vi "autofocus calibrate.vi"() -> ()   [LabVIEW 2014]
uses:
  autofocus-globals.vi
  Stage Control/Stage SubVis/move stage.ctl
panel:
  out "Calibration curve":cluster{dbl[], ext[]}(graph)
  out "Cal. curve":cluster{ext[], dbl[]}
  out "Intensity OK":bool=TRUE
  in  "Error In":errorcluster
  out "Error Out":errorcluster
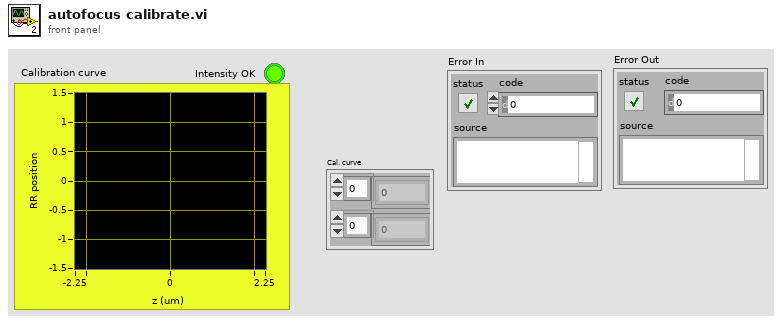
[diagram p1: front panel]
types:
  T1 = typedef "move stage.ctl" = cluster{"dx (um) (0 -> ignore)":ext, "dy (um) (0 -> ignore)":ext, "dz (um) (0 -> ignore)":ext, "Re-center x,y":bool, "Re-center z":bool, "x (um) (-1 -> ignore)":dbl, "y (um) (-1 -> ignore)":dbl, "z (um) (-1 -> ignore)":dbl}
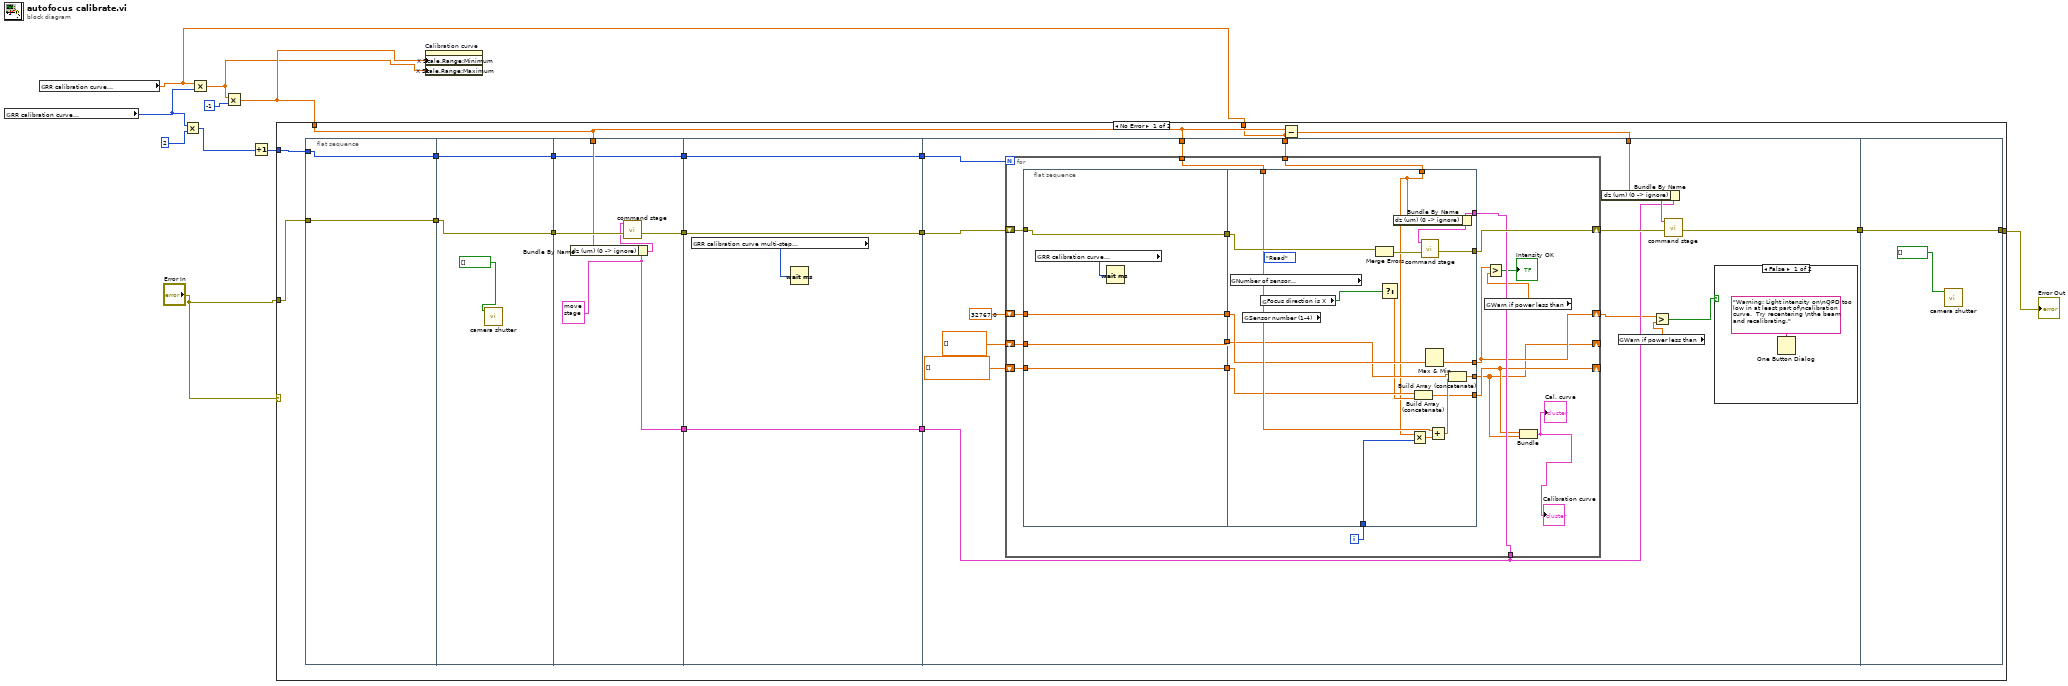
[diagram p0: block diagram]
diagram:
  n1 = global read "autofocus-globals.vi" "RR calibration curve\nhalf-width  (steps)"() -> (w6:u16)
  n2 = global read "autofocus-globals.vi" "RR calibration curve\nstep size (um)"() -> (w3:ext)
  n3 = Multiply(x=w6, y=2) -> (x*y=w5:i32)
  n4 = Multiply(x=w3, y=w6) -> (x*y=w1:ext)
  n5 = Multiply(x=w1, y=-1) -> (x*y=w2:ext)
  n6 = Increment(x=w5) -> (x+1=w4:i32)
  n7 = case shown="No Error" "Error In" {
    tunnel: "Error In" -> [w25 w103]
    tunnel: [w11 w103] -> w9
    tunnel: w2 -> [w15 _]
    tunnel: w4 -> [w27 _]
    tunnel: w3 -> [w14 _]
    frame No Error {
      n8 = flat-sequence {
        tunnel: w27 -> [w28]
        tunnel: [w29] -> w26
        tunnel: w25 -> [w29]
        tunnel: [w28] -> w19
        tunnel: w26 -> [w31]
        tunnel: [w31] -> w24
        tunnel: [w30] -> w20
        tunnel: w19 -> [w30]
        tunnel: w24 -> [w38]
        tunnel: w15 -> [w36]
        tunnel: [w37] -> w23
        tunnel: [w34] -> w22
        tunnel: [w33] -> w21
        tunnel: w20 -> [w33]
        tunnel: w23 -> [w42]
        tunnel: w22 -> [w41]
        tunnel: w21 -> [w39]
        tunnel: [w42] -> w18
        tunnel: [w41] -> w17
        tunnel: [w39] -> w16
        tunnel: w18 -> [w56]
        tunnel: w17 -> [w47]
        tunnel: w16 -> [w57]
        tunnel: w15 -> [w52]
        tunnel: w14 -> [w51]
        tunnel: w13 -> [w49]
        tunnel: [w46] -> w12
        tunnel: [w102] -> w11
        tunnel: w12 -> [w102]
        frame #0 {
        }
        frame #1 {
          n9 = call "camera shutter.vi"("Array"=bool[] []) -> ()  [unwired: 10 in, 1 out]
        }
        frame #2 {
          w34 = T1 {"dx (um) (0 -> ignore)"=0.0, "dy (um) (0 -> ignore)"=0.0, "dz (um) (0 -> ignore)"=0.0, "Re-center x,y"=FALSE, "Re-center z"=FALSE, "x (um) (-1 -> ignore)"=-1.0, "y (um) (-1 -> ignore)"=-1.0, "z (um) (-1 -> ignore)"=-1.0} ("Command Stage")
          n10 = Bundle By Name(cluster=w34, "dz (um) (0 -> ignore)"=w36) -> (w35:T1)
          n11 = call "command stage.vi"("Error In"=w38, "Command Stage"=w35) -> ("Error Out"=w37:errorcluster)  [unwired: 9 in]
        }
        frame #3 {
          n12 = global read "autofocus-globals.vi" "RR calibration curve multi-step\nadd'l settle time (ms)"() -> (w40:u16)
          n13 = Wait (ms)(milliseconds to wait=w40) -> ()  [unwired: 1 out]
        }
        frame #4 {
          n14 = for {
            N: w57 -> [_]
            shift-right: [w69] -> w50
            shift-left: w56 -> [w77]
            shift-right: [w62] -> w45
            shift-left: 32767.0 -> [w73]
            shift-right: [w60] -> _
            shift-left: dbl[] [] ("z (um)") -> [w74]
            shift-right: [w61] -> _
            shift-left: dbl[] [] ("QPD position") -> [w75]
            tunnel: w52 -> [w68]
            tunnel: w51 -> [w66]
            tunnel: w47 -> [w65]
            i -> [w67]
            n15 = flat-sequence {
              tunnel: w77 -> [w81]
              tunnel: [w81] -> w76
              tunnel: w75 -> [w80]
              tunnel: w74 -> [w79]
              tunnel: w73 -> [w78]
              tunnel: [w80] -> w72
              tunnel: [w79] -> w71
              tunnel: [w78] -> w70
              tunnel: w76 -> [w100]
              tunnel: w72 -> [w90]
              tunnel: w71 -> [w91]
              tunnel: w70 -> [w93]
              tunnel: [w95] -> w69
              tunnel: w68 -> [w94]
              tunnel: [w92] -> w62
              tunnel: [w88] -> w61
              tunnel: w67 -> [w87]
              tunnel: w66 -> [w86]
              tunnel: w65 -> [w85]
              tunnel: [w83] -> w60
              frame #0 {
                n16 = global read "autofocus-globals.vi" "RR calibration curve\nsettle time (ms)"() -> (w82:u16)
                n17 = Wait (ms)(milliseconds to wait=w82) -> ()  [unwired: 1 out]
              }
              frame #1 {
                (unwired) enum16{"Start", "Read", "End"}."Read" ("Mode")
                n18 = global read "autofocus-globals.vi" "Number of sensor\nreadings to average"() -> ()  [unwired: 1 out]
                n19 = global read "autofocus-globals.vi" "Sensor number (1-4)"() -> ()  [unwired: 1 out]
                n20 = global read "autofocus-globals.vi" "Focus direction is X"() -> (w84:bool)
                n21 = Merge Errors(w100) -> (w99:errorcluster)  [unwired: 1 in]
                n22 = Select(s=w84) -> (s? t:f=w89:dbl)  [unwired: 2 in]
                n23 = Bundle By Name(cluster=w85, "dz (um) (0 -> ignore)"=w86) -> ()  [unwired: 1 out]
                n24 = Multiply(x=w86, y=w87) -> (x*y=w98:ext)
                n25 = Build Array (concatenate)(w90, w89) -> (w88:dbl[])
                n26 = call "command stage.vi"("Error In"=w99, "Command Stage"=w85) -> ("Error Out"=w95:errorcluster)  [unwired: 9 in]
                n27 = Max & Min(y=w93) -> (x=w96:dbl, min(x,y)=w92:dbl)  [unwired: 1 out]
                n28 = Add(x=w94, y=w98) -> (x+y=w97:ext)
                n29 = Build Array (concatenate)(w91, w97) -> (w83:ext[])
              }
            }
            n30 = global read "autofocus-globals.vi" "Warn if power less than"() -> (w63:dbl)
            n31 = Greater?(x=w62, y=w63) -> (0:→"Intensity OK":bool)
            n32 = Bundle(w61, w60) -> (→"Cal. curve" →"Calibration curve":cluster{dbl[], ext[]})  [unwired: 1 in]
          }
          n33 = Bundle By Name(cluster=w47, "dz (um) (0 -> ignore)"=w49) -> (w48:T1)
          n34 = global read "autofocus-globals.vi" "Warn if power less than"() -> (w44:dbl)
          n35 = Greater?(x=w45, y=w44) -> (0:w43:bool)
          n36 = call "command stage.vi"("Error In"=w50, "Command Stage"=w48) -> ("Error Out"=w46:errorcluster)  [unwired: 9 in]
          n37 = case shown="False" w43 {
            frame False {
              n38 = One Button Dialog(message="Warning: Light intensity on\nQPD too low in at least part of\ncalibration curve.  Try recentering \nthe beam and recalibrating.") -> ()  [unwired: 2 out]
            }
            frame True {
            }
          }
        }
        frame #5 {
          n39 = call "camera shutter.vi"("Array"=bool[] []) -> ()  [unwired: 10 in, 1 out]
        }
      }
      n40 = Subtract(x=w15, y=w14) -> (x-y=w13:ext)
    }
    frame Error {
    }
  }
  "Error Out" <- w9
  n41 = property on="Calibration curve" class="XYGraph (strict)"("X Scale.Range:Minimum"=w2, "X Scale.Range:Maximum"=w1) -> ()  [unwired: 2 in, 2 out]
